vi "Create SubChannels for CIPC Cluster.vi"(11 "Buffer Configuration":T1) -> (3 "SubChannels for OOB":refnum<class "CIFChannels.lvclass">[](array[class]))   [LabVIEW 2021, in "CIFChannelMng.lvclass"]
doc: "This utility will advertize the individual channels of a CIPC cluster. The override name needs to be the name of the original CICP channel. This is what the subscribers connect for reading data. The individual elements are read using the type and offset to only read a single element."
uses:
  CIFChannelMng.lvclass
  CIFChannelMng.lvclass/CIFChannelMng.ctl
  <vilib>/CIF Foundation/CIF CIPC/CIF_NI_CIPC.lvlib
  <vilib>/CIF Foundation/CIF Channels Core/CIFChannels/CIFChannels.lvclass
  <vilib>/CIF Foundation/CIF Channels Core/ChannelCommon/typedef/Channel State.ctl
  <vilib>/CIF Foundation/CIF Channels Core/ChannelCommon/ChannelCommon.lvlib
  <vilib>/CIF Foundation/CIF Channels Core/ChannelCommon/typedef/Direction.ctl
  <vilib>/CIF Foundation/CIF Channels Core/ChannelCommon/typedef/Channel Pattern.ctl
  <vilib>/CIF Foundation/CIF Channels Core/CIPC_Channels/CIF_CIPC_Chan/CIF_CIPC_Chn.lvclass
  <vilib>/CIF Foundation/CIF Channels Core/CIPC_Channels/I64/CIF_CIPC_Chn_I64.lvclass
  <vilib>/CIF Foundation/CIF Channels Core/CIPC_Channels/U64/CIF_CIPC_Chn_U64.lvclass
  <vilib>/CIF Foundation/CIF Channels Core/CIPC_Channels/Double/CIF_CIPC_Chn_Double.lvclass
  C:/Program Files/National Instruments/LabVIEW 2021/vi.lib/CIF Foundation/CIF Channels Core/CIPC_Channels/CIF_CIPC_Chan/CIF_CIPC_Chn.lvclass
  C:/Program Files/National Instruments/LabVIEW 2021/vi.lib/CIF Foundation/CIF Channels Core/CIFChannels/CIFChannels.lvclass
  C:/Program Files/National Instruments/LabVIEW 2021/vi.lib/CIF Foundation/CIF Channels Core/CIPC_Channels/I64/CIF_CIPC_Chn_I64.lvclass
  C:/Program Files/National Instruments/LabVIEW 2021/vi.lib/CIF Foundation/CIF Channels Core/CIPC_Channels/U64/CIF_CIPC_Chn_U64.lvclass
  C:/Program Files/National Instruments/LabVIEW 2021/vi.lib/CIF Foundation/CIF Channels Core/CIPC_Channels/Double/CIF_CIPC_Chn_Double.lvclass
  <vilib>/CIF Foundation/CIF Channels Core/CIPC_Channels/CIF_CIPC_Chan/Typedef/Buffer Configuration Data.ctl
  <vilib>/CIF Foundation/CIF CIPC/TypeDefs/Backpressure References.ctl
  <vilib>/CIF Foundation/CIF CIPC/TypeDefs/Backpressure Names.ctl
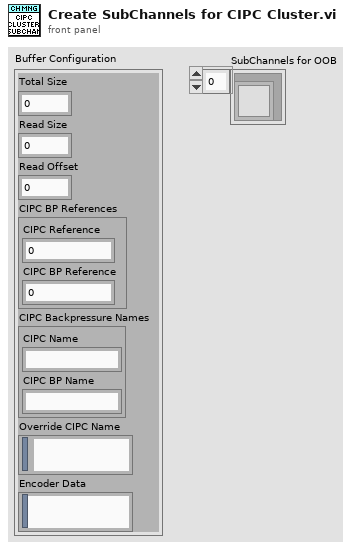
[diagram p1: front panel]
types:
  T1 = typedef "CIF_CIPC_Chn.lvclass/Buffer Configuration Data.ctl" = cluster{"Total Size":u32, "Read Size":u32, "Read Offset":u32, "CIPC BP References":T2, "CIPC Backpressure Names":T3, "Override CIPC Name":string, "Encoder Data":string}
  T2 = typedef "CIF_NI_CIPC.lvlib/Backpressure References.ctl" = cluster{"CIPC Reference":u64, "CIPC BP Reference":u64}
  T3 = typedef "CIF_NI_CIPC.lvlib/Backpressure Names.ctl" = cluster{"CIPC Name":string, "CIPC BP Name":string}
  T4 = typedef "CIF_NI_CIPC.lvlib/Data Encoding.ctl" = cluster{"Data Struct Info":cluster{"Alignment":T5, "Endian":T6, "Array Info":T7, "Total Length (bytes)":i32}, "Data Elements":T8[]}
  T5 = typedef "CIF_NI_CIPC.lvlib/Alignment.ctl" = enum16{"Natural", "Packed"}
  T6 = typedef "DataTypes_CIF_U.lvlib/Endian.ctl" = enum16{"Little Endian", "Big Endian"}
  T7 = typedef "CIF_NI_CIPC.lvlib/Data Struct Array Info.ctl" = cluster{"Array":bool, "Array_Size":i32, "Elem_Size":i32, "Prepended Length":bool}
  T8 = typedef "CIF_NI_CIPC.lvlib/Data Element.ctl" = cluster{"Name":string, "Type":T9, "Size":u32, "Offset":u32}
  T9 = typedef "NI_Data Type.lvlib/Data Type.ctl" = enum8{"Invalid Type", "Void", "I8", "I16", "I32", "I64", "U8", "U16", "U32", "U64", "Single Float", "Double Float", "Extended Float", "Single Complex", "Double Complex", "Extended Complex", "Enum U8", "Enum U16", "Enum U32", "Enum U64", "Single Float With Unit", "Double Float With Unit", "Extended Float With Unit", "Single Complex with Unit", "Double Complex with Unit", "Extended Complex with Unit", "Boolean", "String", "Path", "Picture", "Tag", "Array", "Cluster", "Variant", "LV Variant", "Waveform", "Timestamp", "Digital Waveform", "Digital Data", "ExpressData", "Refnum", "External Data", "VI", "Poly VI", "LabVIEW Class Instance", "Fixed Point", "Set Collection", "Map Collection"}
  T10 = typedef "ChannelCommon.lvlib/Channel Pattern.ctl" = enum8{"Unknown", "Tag", "FIFO", "MultiFIFO", "BackpressureFIFO"}
  T11 = typedef "ChannelCommon.lvlib/Direction.ctl" = enum8{"Publisher", "Subscriber"}
  T12 = typedef "ChannelCommon.lvlib/Channel State.ctl" = enum8{"Creating", "Disconnected", "Connecting", "Connected", "Destroyed"}
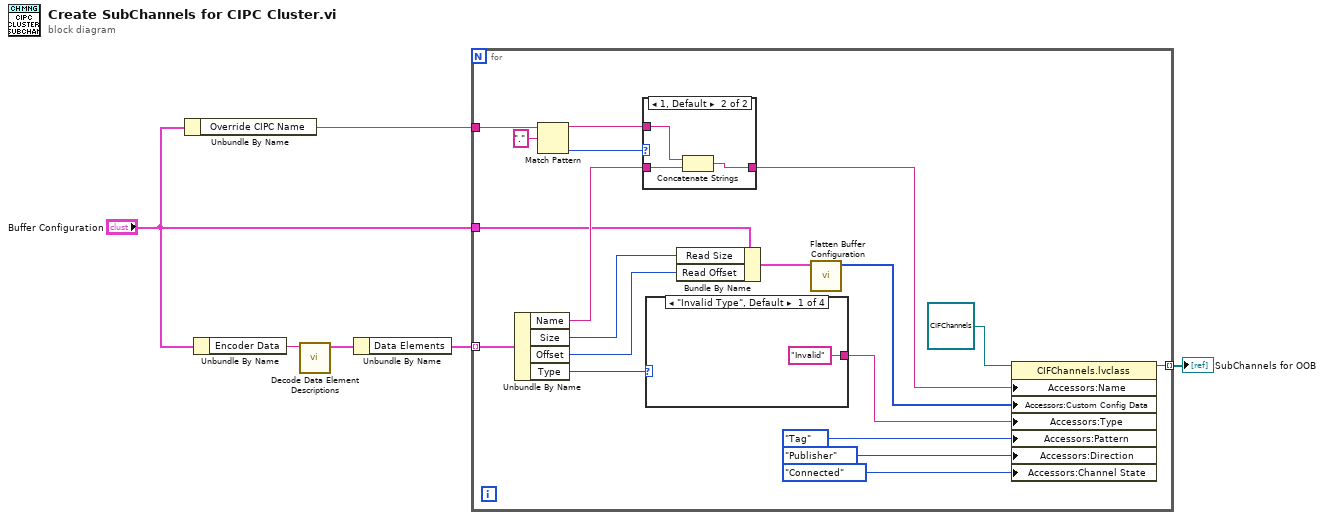
[diagram p0: block diagram]
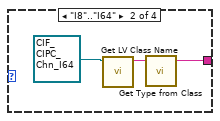
[diagram p3: hidden frame]
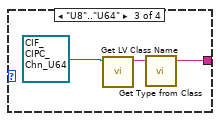
[diagram p4: hidden frame]
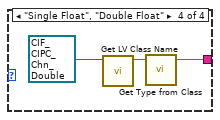
[diagram p5: hidden frame]
diagram:
  n1 = Unbundle By Name("Buffer Configuration") -> ("Override CIPC Name"=w6:string)
  n2 = Unbundle By Name("Buffer Configuration") -> ("Encoder Data"=w4:string)
  n3 = call <vilib>:"Decode Data Element Descriptions.vi"("Encoder Data Description"=w4) -> ("Data Encoding"=w2:T4)  [unwired: 10 in]
  n4 = Unbundle By Name(w2) -> ("Data Elements"=w1:T8[])
  n5 = for {
    tunnel: w6 -> [w11]
    tunnel: "Buffer Configuration" -> [w9]
    tunnel: w1 -> [w8] mode=indexing
    tunnel: [w7] -> w3 mode=indexing
    n6 = Unbundle By Name(w8) -> ("Name"=w17:string, "Size"=w13:u32, "Offset"=w12:u32, "Type"=w21:T9)
    n7 = Match Pattern(string=w11, regular expression=".") -> (before substring=w18:string, offset past match=w10:i32)  [unwired: 1 in, 2 out]
    n8 = case shown="1, Default" w10 {
      tunnel: w18 -> [_ w29]
      tunnel: w17 -> [w26 w27]
      tunnel: [w26 w28] -> w16
      frame -1 {
      }
      frame 1, Default {
        n9 = Concatenate Strings(w29, w27) -> (w28:string)
      }
    }
    n10 = case shown="\"Invalid Type\", Default" w21 {
      tunnel: ["Invalid" ("Channel Type") w31 w35 w38] -> w20
      frame "Invalid Type", Default {
      }
      frame "I8".."I64" {
        n11 = call <vilib>:"Get LV Class Name.vi"("object"=refnum<class "CIF_CIPC_Chn_I64.lvclass"> refnum ("CIFTag in")) -> ("class name"=w33:string)  [unwired: 9 in, 1 out]
        n12 = call <vilib>:"Get Type from Class.vi"("Class"=w33) -> ("Channel Type"=w31:string)  [unwired: 4 in]
      }
      frame "U8".."U64" {
        n13 = call <vilib>:"Get LV Class Name.vi"("object"=refnum<class "CIF_CIPC_Chn_U64.lvclass"> refnum ("CIFTag in")) -> ("class name"=w36:string)  [unwired: 9 in, 1 out]
        n14 = call <vilib>:"Get Type from Class.vi"("Class"=w36) -> ("Channel Type"=w35:string)  [unwired: 4 in]
      }
      frame "Single Float", "Double Float" {
        n15 = call <vilib>:"Get LV Class Name.vi"("object"=refnum<class "CIF_CIPC_Chn_Double.lvclass"> refnum ("CIFTag in")) -> ("class name"=w39:string)  [unwired: 9 in, 1 out]
        n16 = call <vilib>:"Get Type from Class.vi"("Class"=w39) -> ("Channel Type"=w38:string)  [unwired: 4 in]
      }
    }
    n17 = Bundle By Name(cluster=w9, "Read Size"=w13, "Read Offset"=w12) -> (w15:T1)
    n18 = call <vilib>:"Flatten Buffer Configuration.vi"("Buffer Configuration"=w15) -> ("Flattened Configuration"=w14:u8[])  [unwired: 10 in]
    n19 = property class="CIFChannels.lvclass"(reference=refnum<class "CIFChannels.lvclass"> refnum, "Accessors:Name"=w16, "Accessors:Custom Config Data"=w14, "Accessors:Type"=w20, "Accessors:Pattern"=Channel_Pattern."Tag" ("Pattern"), "Accessors:Direction"=Direction."Publisher" ("Direction"), "Accessors:Channel State"=Channel_State."Connected" ("Channel State")) -> (reference out=w7:refnum<class "CIFChannels.lvclass">)  [unwired: 1 in, 1 out]
  }
  "SubChannels for OOB" <- w3
